vi "Delete Empty Array.vi"(8 "error in":errorcluster, 11 "Array in":string[](array[string])) -> (0 "error out":errorcluster, 3 "Array out":string[](array[string]))   [LabVIEW 2018]
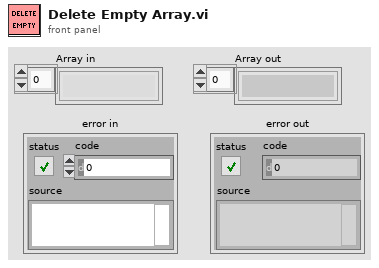
[diagram p1: front panel]
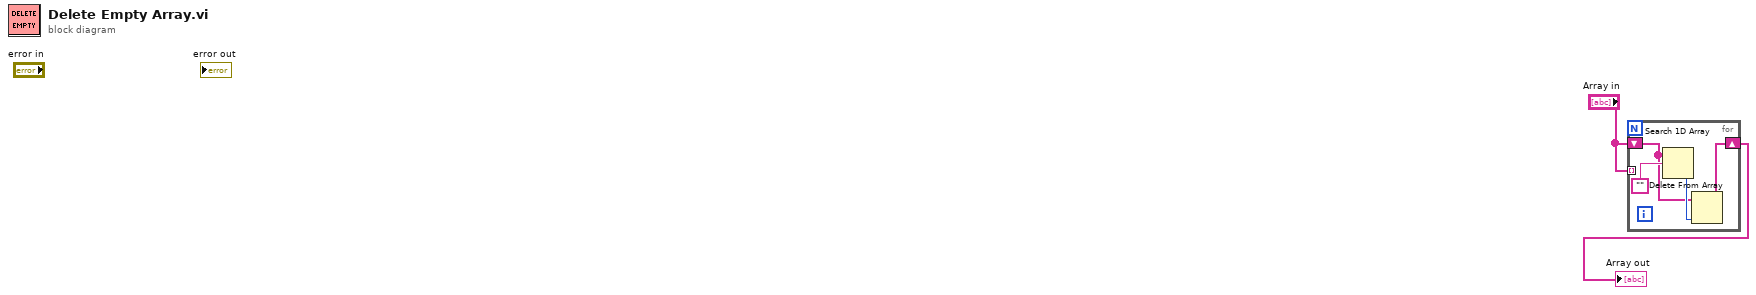
[diagram p0: block diagram]
diagram:
  n1 = for {
    tunnel: "Array in" -> [_] mode=indexing
    shift-right: [w4] -> w1
    shift-left: "Array in" -> [w3]
    n2 = Search 1D Array(1D array=w3, element="") -> (index of element=w5:i32)  [unwired: 1 in]
    n3 = Delete From Array(array=w3, index=w5) -> (array with subset deleted=w4:string[])  [unwired: 1 in, 1 out]
  }
  "Array out" <- w1
